vi "Fdx Get Tx Queue Status.vi"(8 "error in (no error)":errorcluster, 11 "InstrumentHandle in":u32) -> (0 "error out":errorcluster, 1 "TxQueueStatus":T1 {"QueueStatus" items=["FDX_QUE_EMPTY", "FDX_QUE_FILLED", "FDX_QUE_FULL", "FDX_QUE_SENT", "FDX_QUE_CYCL_RUN", "FDX_QUE_CYCL_SENT"]}, 3 "InstrumentHandle out":u32)   [LabVIEW 2020, in "AIM664LV.lvlib"]
uses:
  AIM664LV.lvlib
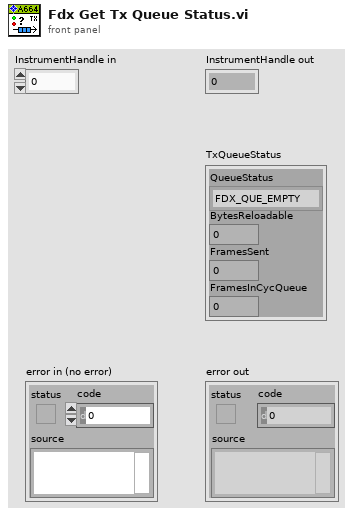
[diagram p1: front panel]
types:
  T1 = cluster{"QueueStatus":i32, "BytesReloadable":u32, "FramesSent":u32, "FramesInCycQueue":u32}
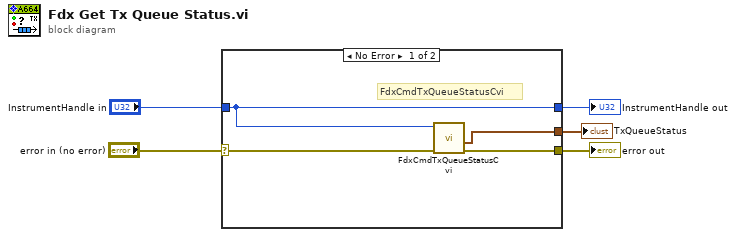
[diagram p0: block diagram]
diagram:
  n1 = case shown="No Error" "error in (no error)" {
    selector: "error in (no error)" -> [w9 w10]
    tunnel: "InstrumentHandle in" -> [w6 w11]
    tunnel: [w8 w10] -> w3
    tunnel: [w6 w11] -> w2
    tunnel: [w7 _] -> w1
    frame No Error {
      # "FdxCmdTxQueueStatusCvi"
      n2 = call "FdxCmdTxQueueStatusCvi.vi"("error in"=w9, "InstrumentHandle"=w6) -> ("error out"=w8:errorcluster, "TxQueueStatus"=w7:T1)  [unwired: 7 in, 1 out]
    }
    frame Error {
    }
  }
  "error out" <- w3
  "InstrumentHandle out" <- w2
  "TxQueueStatus" <- w1
